vi "Teardown.vi"(11 "Base Queue Actor in":refnum<class "Base Queue Actor.lvclass">) -> (3 "Base Queue Actor out":refnum<class "Base Queue Actor.lvclass">)   [LabVIEW 2021, in "jettl.lvlib" / "Base Queue Actor.lvclass"]
uses:
  Base Queue Actor.lvclass
  Queue State/Teardown Queue State/Teardown Queue State.lvclass
  C:/git/jettl/src/jettl/Queue State/Queue State/Queue State.lvclass
  Base Queue Actor.lvclass/Base Queue Actor.ctl
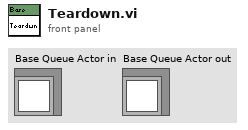
[diagram p1: front panel]
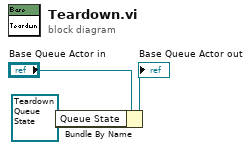
[diagram p0: block diagram]
diagram:
  n1 = Bundle By Name(cluster="Base Queue Actor in", "Queue State"=refnum<class "Teardown Queue State.lvclass"> refnum ("jettl.lvlib:Teardown Queue State.lvclass")) -> (→"Base Queue Actor out":refnum<class "Base Queue Actor.lvclass">)
